vi "AssertVIExecRunning.vi"(0 "VI Reference In":refnum<vi>, 1 "Test Label":string, 3 "Assert Only? (F)":bool, 11 "Error In":errorcluster, 12 "Assert Interval(10 ms)":u32=10, 13 "Timeout(5 sec)":dbl=5.0) -> (4 "VI Reference Out":refnum<vi>, 6 "Asserted Value":T1(ring), 15 "Error Out":errorcluster)   [LabVIEW 2016, in "Drona.lvlib" / "AssertVI.lvlib"]
doc: "Asserts if the VI is in Running state.\nThe input control name is given as a string , incase of path, use delimiters inbetween the path."
uses:
  AssertVI.lvlib
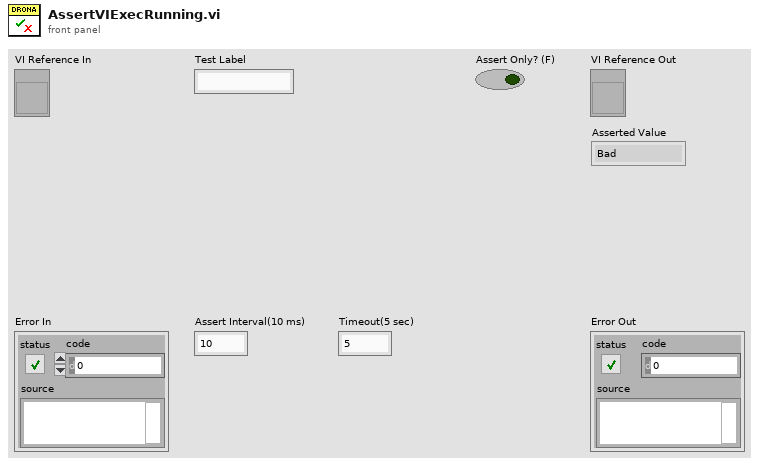
[diagram p1: front panel]
types:
  T1 = enum32{"Bad", "Idle", "Run top level", "Running"}
  T2 = enum32{"Bad", "Idle", "Run top level", "Running"}[]
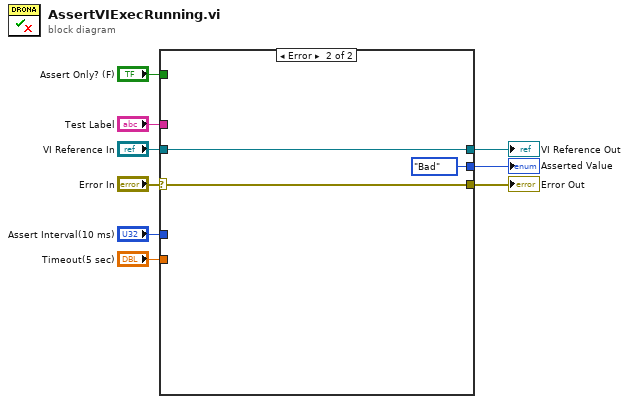
[diagram p0: block diagram]
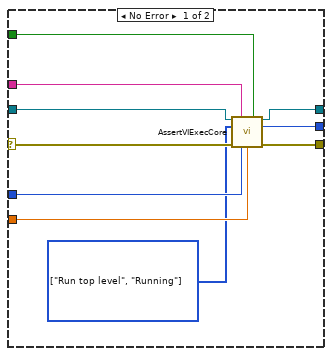
[diagram p2: hidden frame]
diagram:
  n1 = case shown="Error" "Error In" {
    selector: "Error In" -> [w18 w22]
    tunnel: [w19 w22] -> w9
    tunnel: "Timeout(5 sec)" -> [w17 _]
    tunnel: [w16 w21] -> w6
    tunnel: "Assert Interval(10 ms)" -> [w15 _]
    tunnel: "Test Label" -> [w14 _]
    tunnel: "VI Reference In" -> [w13 w21]
    tunnel: "Assert Only? (F)" -> [w12 _]
    tunnel: [w10 T1."Bad" ("Asserted Value")] -> w1
    frame No Error {
      w11 = T2 [enum."Run top level", enum."Running"] items=["Bad", "Idle", "Run top level", "Running"] ("Execution:State")
      n2 = call "AssertVIExecCore.vi"("VI Reference In"=w13, "Label"=w14, "Assert Only? (F)"=w12, "Execution:State"=w11, "Error In"=w18, "Assert Interval(10 ms)"=w15, "Timeout(5 sec)"=w17) -> ("VI Reference Out"=w16:refnum<vi>, "Asserted Value"=w10:T1, "Error Out"=w19:errorcluster)  [unwired: 6 in]
    }
    frame Error {
    }
  }
  "Error Out" <- w9
  "VI Reference Out" <- w6
  "Asserted Value" <- w1
